vi "Write Size.vi"(8 "error in (no error)":errorcluster, 10 "Size":T1, 11 "MulticolumnListbox.lvclass in":refnum<class "MulticolumnListbox.lvclass">) -> (0 "error out":errorcluster, 3 "MulticolumnListbox.lvclass out":refnum<class "MulticolumnListbox.lvclass">)   [LabVIEW 2015, in "MulticolumnListbox.lvclass"]
uses:
  MulticolumnListbox.lvclass
  <vilib>/Utility/miscctls.llb/LVBoundsTypeDef.ctl
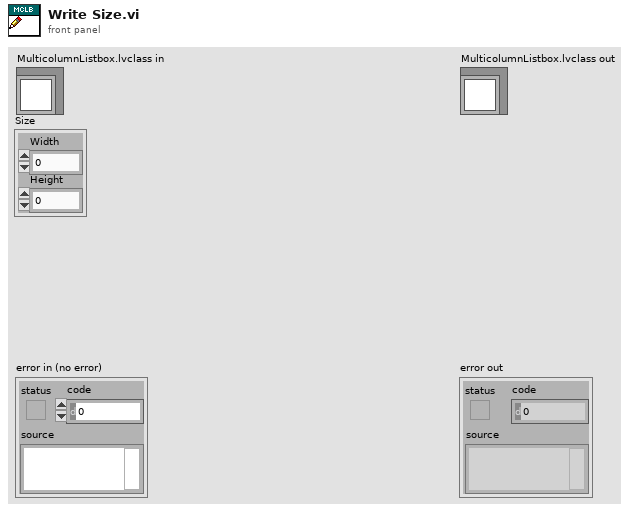
[diagram p1: front panel]
types:
  T1 = typedef "LVBoundsTypeDef.ctl" = cluster{"Width":u32, "Height":u32}
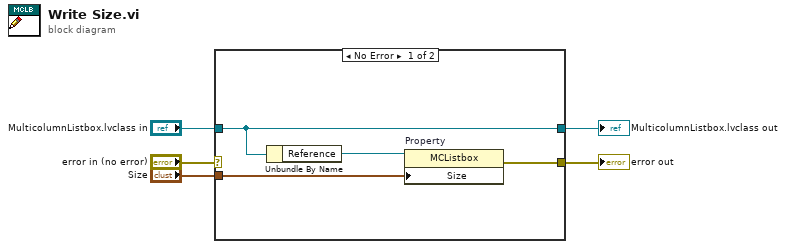
[diagram p0: block diagram]
diagram:
  n1 = case shown="No Error" "error in (no error)" {
    selector: "error in (no error)" -> [_ w11]
    tunnel: [w9 w11] -> w4
    tunnel: [w7 w10] -> w2
    tunnel: "MulticolumnListbox.lvclass in" -> [w7 w10]
    tunnel: "Size" -> [w8 _]
    frame No Error {
      n2 = Unbundle By Name(w7) -> ("Reference"=w6:refnum<vi>)
      n3 = property on="Property" class="MCListbox"(reference=w6, "Size"=w8) -> (error out=w9:errorcluster)  [unwired: 1 in, 1 out]
    }
    frame Error {
    }
  }
  "error out" <- w4
  "MulticolumnListbox.lvclass out" <- w2
